vi "실습 9-1 경로 만들기.vi"() -> ()   [LabVIEW 2014]
panel:
  out "에러 출력":errorcluster
  out "created path":path
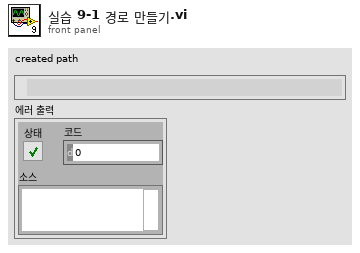
[diagram p1: front panel]
types:
  T1 = enum16{"open", "replace", "create", "open or create", "replace or create", "replace or create with confirmation"}
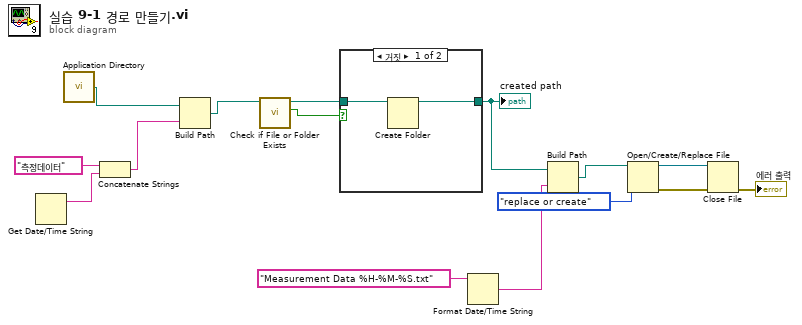
[diagram p0: block diagram]
diagram:
  n1 = Get Date/Time String() -> (date string=w14:string)  [unwired: 3 in, 1 out]
  n2 = call <vilib>:"Application Directory.vi"() -> ("Application Directory"=w12:path)
  n3 = Concatenate Strings("측정데이터" ("문자열"), w14) -> (w13:string)
  n4 = Build Path(base path=w12, name or relative path=w13) -> (appended path=w11:path)
  n5 = call <vilib>:"Check if File or Folder Exists.vi"("path"=w11) -> ("file or folder exists?"=w9:bool, "dup path"=w10:path)  [unwired: 8 in, 1 out]
  n6 = case shown="거짓" w9 {
    tunnel: w10 -> [w17 w18]
    tunnel: [w16 w18] -> w7
    frame False {
      n7 = Create Folder(path (use dialog)=w17) -> (created path=w16:path)  [unwired: 2 in, 2 out]
    }
    frame True {
    }
  }
  "created path" <- w7
  n8 = Format Date/Time String(time format string (%c)="Measurement Data %H-%M-%S.txt" ("시간 포맷 문자열 (%c)")) -> (date/time string=w6:string)  [unwired: 2 in]
  n9 = Build Path(base path=w7, name or relative path=w6) -> (appended path=w5:path)
  n10 = Open/Create/Replace File(file path (use dialog)=w5, operation (0:open)=T1."replace or create" ("동작(0:open)")) -> (refnum out=w3:refnum<file>, error out=w2:errorcluster)  [unwired: 4 in, 1 out]
  n11 = Close File(refnum=w3, error in=w2) -> (error out=→"에러 출력":errorcluster)  [unwired: 1 out]
